vi "Read_Joint_States.vi"(0 "error in":errorcluster, 2 "Units (deg)":enum16{"Radians", "Degrees"}(ring)=enum."Degrees", 3 "node":string) -> (1 "error out":errorcluster, 4 "Joint States":T1(array[cluster]))   [LabVIEW 2010]
doc: "Read all the current joint states (names, positions, velocity, and efforts)"
panel:
  out "Reply":string
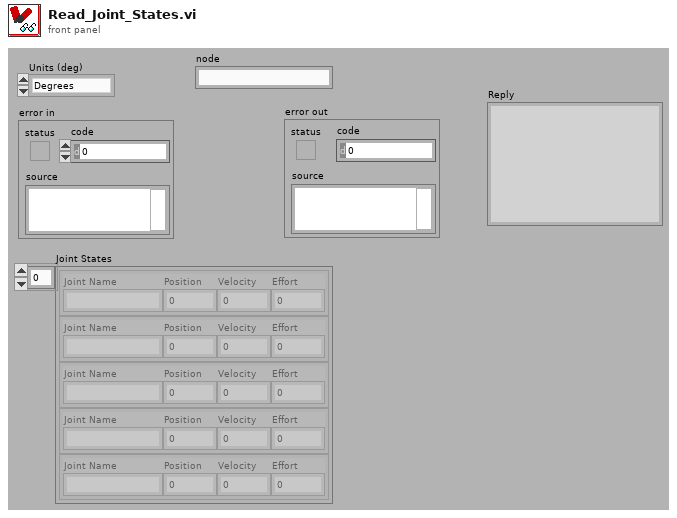
[diagram p1: front panel]
types:
  T1 = cluster{"Joint Name":string, "Position":dbl, "Velocity":dbl, "Effort":dbl}[]
  T2 = typedef "_ROSControl.ctl" = cluster{"topic port":u16, "Node":string, "topic":string, "type":string, "node port":u32, "error ":errorcluster, "Direction":T3, "APIs":string[]}
  T3 = typedef "_ROSDirection.ctl" = enum16{"Node", "Publisher", "Subscriber", "Service Client"}
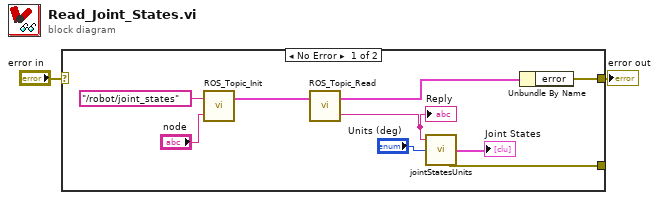
[diagram p0: block diagram]
diagram:
  n1 = case shown="No Error" "error in" {
    selector: "error in" -> [_ w12]
    tunnel: [w11 w12] -> w2
    tunnel: [w6 _] -> _
    frame No Error {
      n2 = call <userlib>:"ROS_Topic_Init.vi"("node"="node", "topic"="/robot/joint_states") -> ("ROS out"=w8:T2)  [unwired: 1 in]
      n3 = call <userlib>:"ROS_Topic_Read.vi"("ROS in"=w8) -> ("Reply"=w3:string, "ROS out"=w7:T2)  [unwired: 1 in]
      "Reply" <- w3
      n4 = call <userlib>:"jointStatesUnits.vi"("Units (deg)"="Units (deg)", "msg in"=w3) -> ("error out"=w6:errorcluster, "Joint States"=→"Joint States":T1)  [unwired: 1 in, 1 out]
      n5 = Unbundle By Name(w7) -> ("error"=w11:errorcluster)
    }
    frame Error {
    }
  }
  "error out" <- w2
